vi "SolenoidSignalBuilder.vi"(0 "Solenoid Status":bool[](array[boolean]), 5 "Pump Status":bool) -> (7 "NI9401_1 Signals":bool[](array[boolean]))   [LabVIEW 2016]
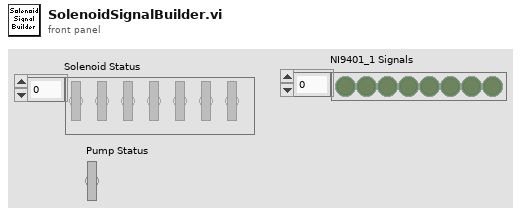
[diagram p1: front panel]
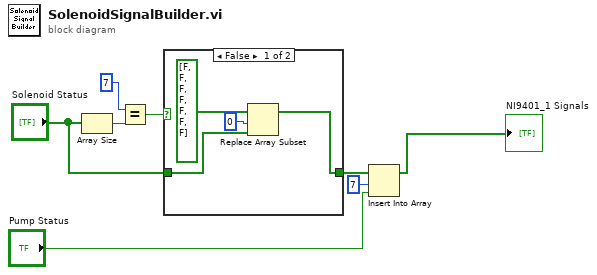
[diagram p0: block diagram]
diagram:
  n1 = Array Size(array="Solenoid Status") -> (size(s)=w8:i32)
  n2 = Equal?(x=7, y=w8) -> (x = y?=w6:bool)
  n3 = case shown="False" w6 {
    tunnel: [w9 w13] -> w2
    tunnel: "Solenoid Status" -> [w11 w13]
    frame False {
      n4 = Replace Array Subset(array=bool[] [FALSE, FALSE, FALSE, FALSE, FALSE, FALSE, FALSE], new element=w11, index=0) -> (w9:bool[])
    }
    frame True {
    }
  }
  n5 = Insert Into Array(array=w2, index=7, new element="Pump Status") -> (→"NI9401_1 Signals":bool[])
